vi "GT Algorithm Find M_ok and J_ok.vi"(8 "Number of Machines":i32=3, 9 "Cmin":u16=25, 10 "Cmin Array":u16[](array[numeric])=[25, 40, 30, 20, 25, 25, 40, 45, 40], 11 "Schedule In":u16[](array[numeric])=[0, 1, 2, 3, 4, 5, 6, 7, 8]) -> (1 "J_ok(Jobs)":i32[](array[numeric]), 2 "M_ok(Machines)":i32[](array[numeric]))   [LabVIEW 2013, in "Scheduler.lvclass"]
uses:
  Scheduler.lvclass
  <userlib>/_OpenG.lib/array/array.llb/Remove Duplicates from 1D Array (I32)__ogtk.vi
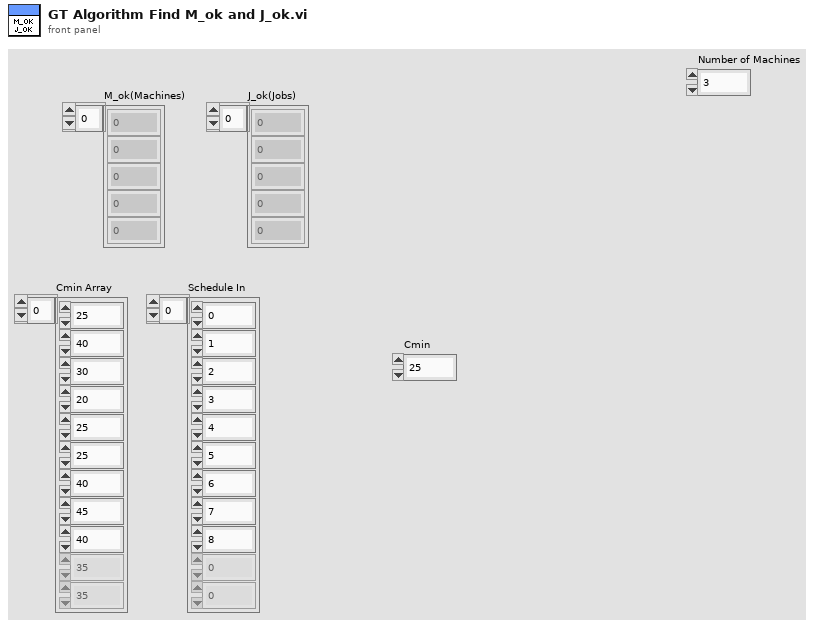
[diagram p1: front panel]
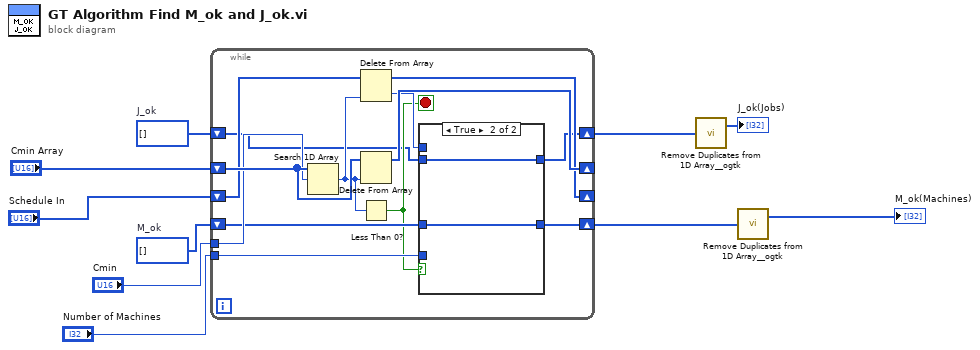
[diagram p0: block diagram]
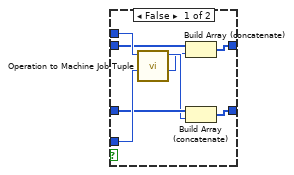
[diagram p2: hidden frame]
diagram:
  w5 = i32[] []  # J_ok
  w6 = i32[] []  # M_ok
  n1 = while {
    shift-right: [w22] -> _
    shift-left: "Cmin Array" -> [w23]
    tunnel: "Cmin" -> [w20]
    tunnel: "Number of Machines" -> [w21]
    shift-right: [w17] -> _
    shift-left: "Schedule In" -> [w18]
    shift-right: [w14] -> w2
    shift-left: w6 -> [w15]
    shift-right: [w11] -> w4
    shift-left: w5 -> [w12]
    stop <- w13 stop-if-true
    n2 = Search 1D Array(1D array=w23, element=w20) -> (index of element=w19:i32)  [unwired: 1 in]
    n3 = Delete From Array(array=w18, index=w19) -> (deleted portion=w16:u16, array with subset deleted=w17:u16[])  [unwired: 1 in]
    n4 = Delete From Array(array=w23, index=w19) -> (array with subset deleted=w22:u16[])  [unwired: 1 in, 1 out]
    n5 = Less Than 0?(x=w19) -> (x < 0?=w13:bool)
    n6 = case shown="True" w13 {
      tunnel: w21 -> [w31 _]
      tunnel: w16 -> [w30 _]
      tunnel: w15 -> [w29 w33]
      tunnel: [w27 w33] -> w14
      tunnel: w12 -> [w26 w32]
      tunnel: [w24 w32] -> w11
      frame False {
        n7 = call "Operation to Machine Job Tuple.vi"("Number of Machines"=w31, "Operation Number"=w30) -> ("Job No"=w25:i32, "Machine No"=w28:i32)  [unwired: 8 in]
        n8 = Build Array (concatenate)(w26, w25) -> (w24:i32[])
        n9 = Build Array (concatenate)(w29, w28) -> (w27:i32[])
      }
      frame True {
      }
    }
  }
  n10 = call-poly <userlib>:"Remove Duplicates from 1D Array__ogtk.vi"("Input Array"=w4) -> ("Output Array"=→"J_ok(Jobs)":i32[])  [unwired: 1 out]
  n11 = call-poly <userlib>:"Remove Duplicates from 1D Array__ogtk.vi"("Input Array"=w2) -> ("Output Array"=→"M_ok(Machines)":i32[])  [unwired: 1 out]
